vi "Test Singleton API.vi"() -> ()   [LabVIEW 2024]
doc: "Singleton API Tester."
uses:
  Singleton.lvlib
  <vilib>/Utility/error.llb/DialogType.ctl
  <vilib>/JKI/JKI Simple Localization/API/JKI Simple LocalizationJKI_Simple_Localization.lvlib
  <vilib>/JKI/JKI Simple Localization/Private/RegisterVIJKI_Simple_Localization.vi
panel:
  in  "NEW EVENT TO HL":bool
  in  "New Event":bool
  in  "Juan":bool caption="Jhon"
  out "last error":errorcluster
  in  "Show Diagram on Init":bool
  in  "wait for reply":bool=TRUE
  in  "Show Block Diagram":bool
  in  "X":dbl=1.0
  out "Reply Payload":dbl
  in  "Stop Module":bool
  in  "Start Module":bool
  out "Do Something Count":i32
  in  "Test Do Something Else and Wait for Reply":bool
  in  "Hide Module Panel":bool
  in  "Show Module Panel":bool
  in  "Test Do Something Else":bool
  in  "Test Do Something":bool
  out "Status":string
  out "Module Running?":bool
  # "This VI tests the API for the Module."
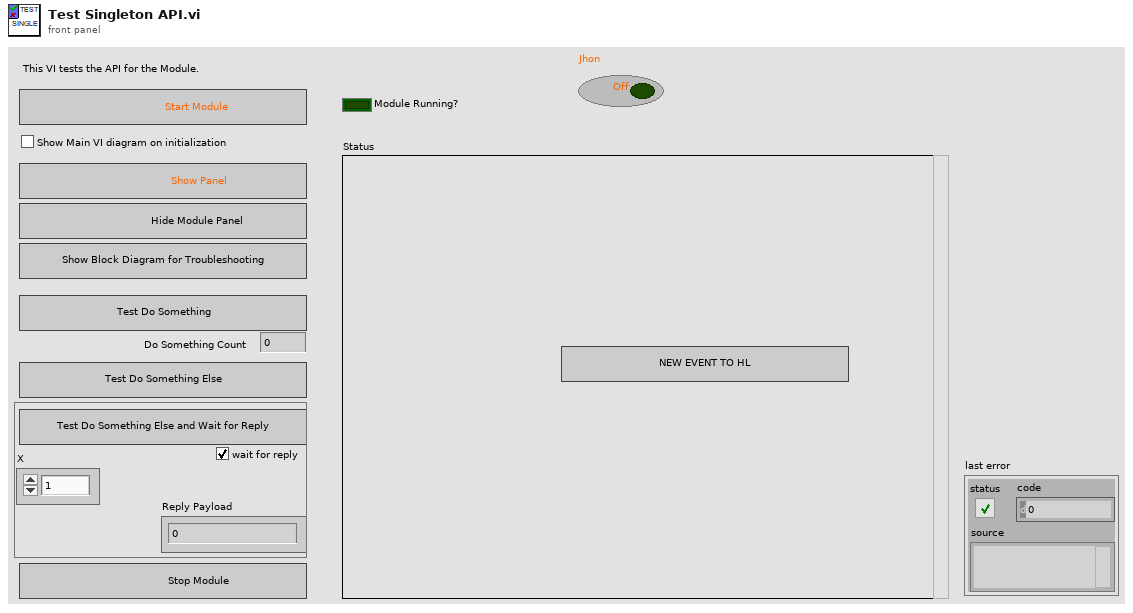
[diagram p1: front panel]
types:
  T1 = typedef "Singleton.lvlib/Broadcast Events--cluster.ctl" = cluster{"Module Did Init":refnum<user-event>, "Status Updated":refnum<user-event>, "Error Reported":refnum<user-event>, "Did Something":refnum<user-event>, "Module Did Stop":refnum<user-event>, "Update Module Execution Status":refnum<user-event>}
  T2 = typedef "DialogType.ctl" = u16
  T3 = typedef "Singleton.lvlib/Do Something Else and Wait (Reply Payload)--cluster.ctl" = cluster{"Value":dbl, "error":errorcluster}
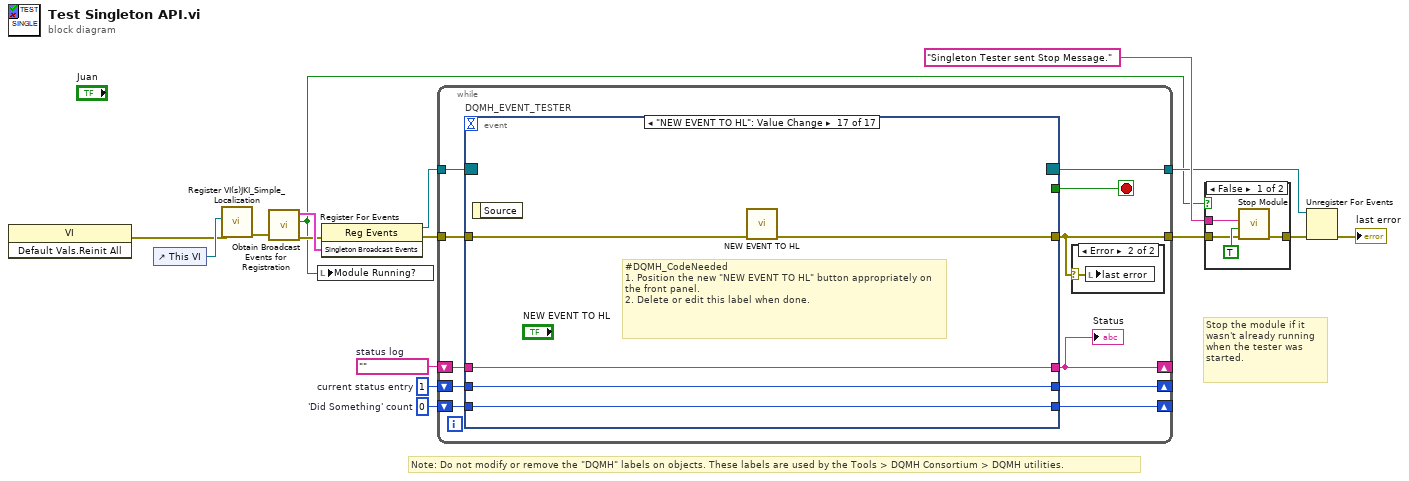
[diagram p0: block diagram]
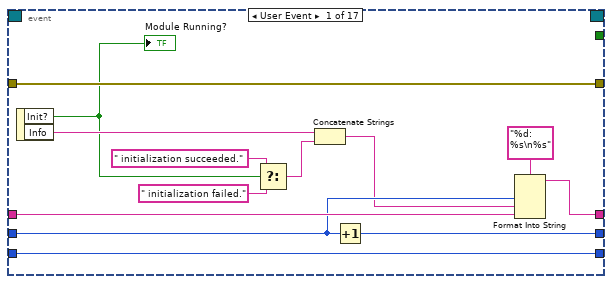
[diagram p4: hidden frame]
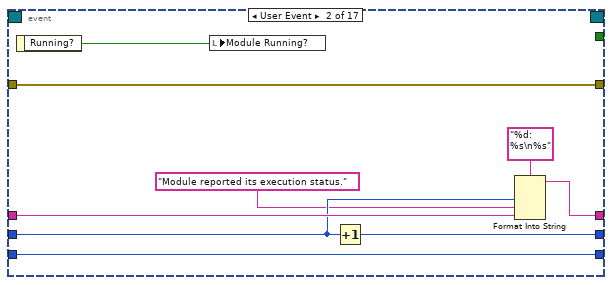
[diagram p5: hidden frame]
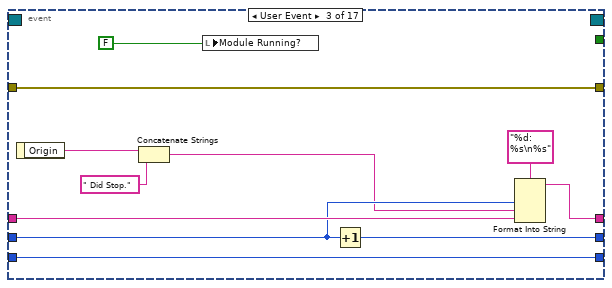
[diagram p6: hidden frame]
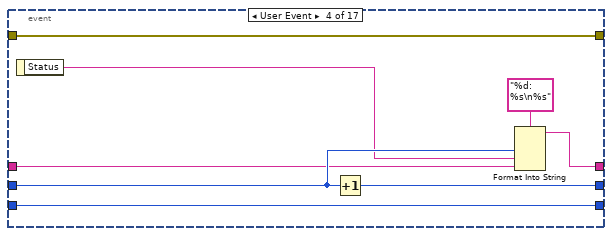
[diagram p7: hidden frame]
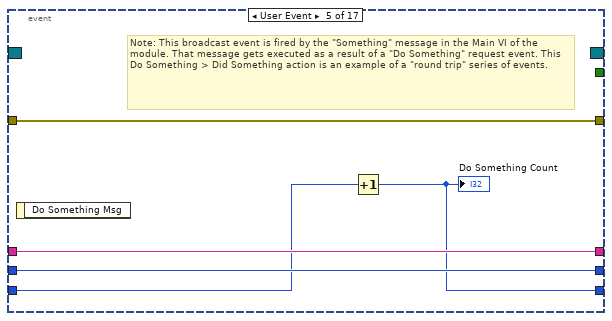
[diagram p8: hidden frame]
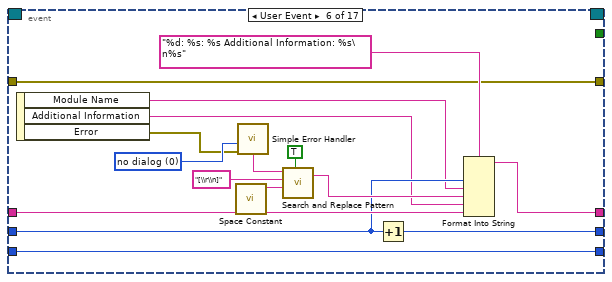
[diagram p9: hidden frame]
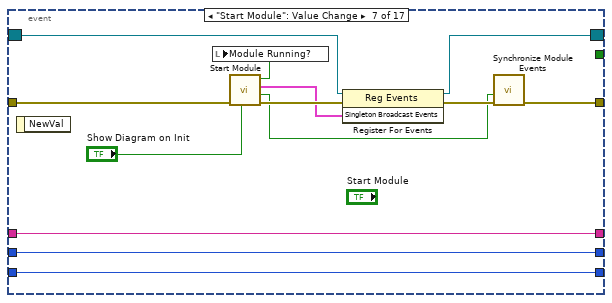
[diagram p10: hidden frame]
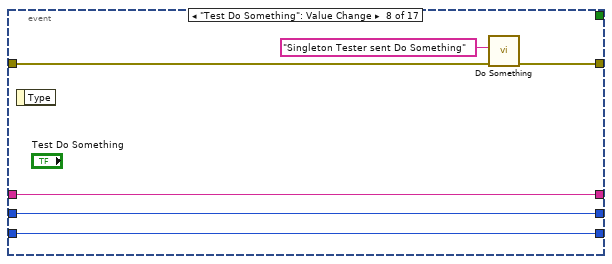
[diagram p11: hidden frame]
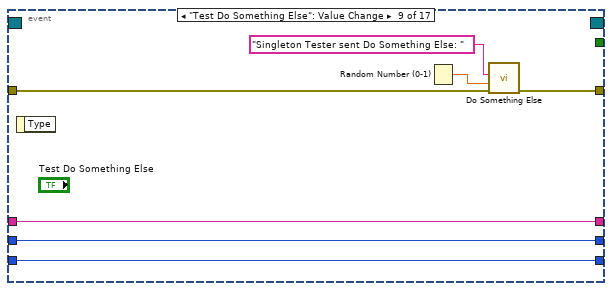
[diagram p12: hidden frame]
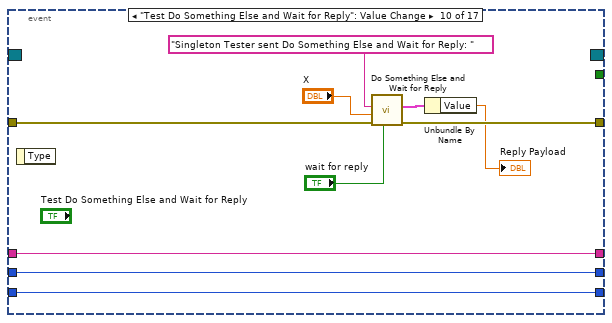
[diagram p13: hidden frame]
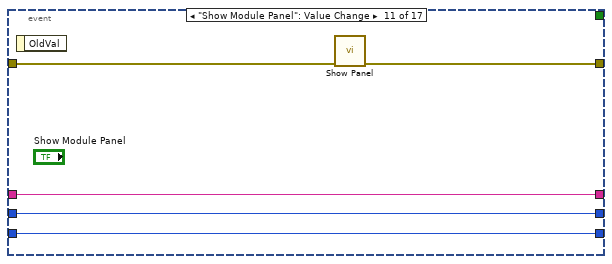
[diagram p14: hidden frame]
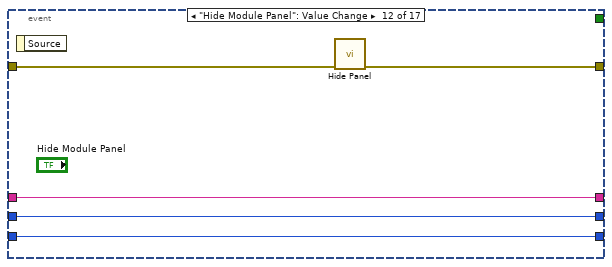
[diagram p15: hidden frame]
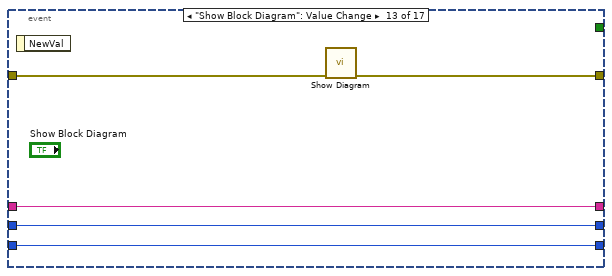
[diagram p16: hidden frame]
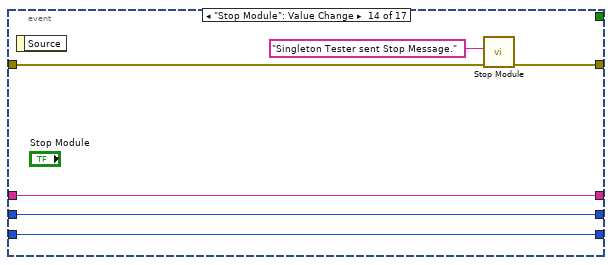
[diagram p17: hidden frame]
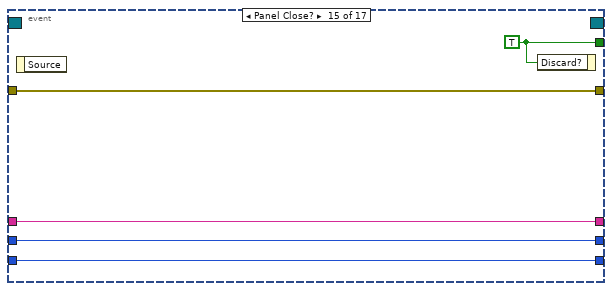
[diagram p18: hidden frame]
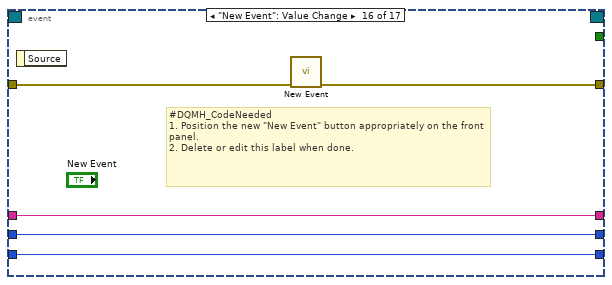
[diagram p19: hidden frame]
diagram:
  w12 = 0  # 'Did Something' count
  w13 = 1  # current status entry
  w14 = ""  # status log
  # "Stop the module if it wasn't already running when the tester was started."
  # "Note: Do not modify or remove the \"DQMH\" labels on objects. These labels are used by the Tools > DQMH Consortium > DQMH utilities."
  n1 = invoke class="VI" method="Default Vals.Reinit All"() -> (error out=w2:errorcluster)  [unwired: 3 in, 2 out]
  n2 = control-ref of="This VI"() -> (w3:refnum<vi>)
  n3 = call-poly <vilib>:"Register VI(s)JKI_Simple_Localization.vi"("error in"=w2, "VI Ref"=w3) -> ("error out"=w1:errorcluster)  [unwired: 8 in, 1 out]
  n4 = call "Obtain Broadcast Events for Registration.vi"("error in"=w1) -> ("error out"=w7:errorcluster, "Already running?"=w6:bool, "Singleton Broadcast Events"=w10:T1)  [unwired: 8 in]
  n5 = local write "Module Running?"(w6) -> ()
  n6 = register-events(error in=w7, w10) -> (reference out=w9:refnum<event-registration>, error out=w11:errorcluster)  [unwired: 1 in]
  n7 = while {
    tunnel: w9 -> [w27]
    tunnel: [w17] -> w5
    shift-right: [w23] -> _
    shift-left: w14 -> [w25]
    shift-right: [w24] -> _
    shift-left: w13 -> [w26]
    shift-right: [w21] -> _
    shift-left: w12 -> [w22]
    tunnel: w11 -> [w20]
    tunnel: [w19] -> w8
    stop <- w18 stop-if-true
    n8 = event "DQMH_EVENT_TESTER" shown="[16] \"NEW EVENT TO HL\": Value Change" {
      selector: w27 -> [_ _ _ _ _ _ w96 _ _ _ _ _ _ _ _ _ _]
      dyn-events: [_ _ _ _ _ _ w95 _ _ _ _ _ _ _ _ _ _] -> w19
      timeout: _ -> [_ _ _ _ _ _ _ _ _ _ _ _ _ _ _ _ _]
      tunnel: [_ _ _ _ _ _ _ _ _ _ _ _ _ _ w152 _ _] -> w18
      tunnel: [w41 w43 w51 w62 w70 w78 w94 w109 w116 w126 w131 w136 w137 w144 w148 w153 w158] -> w17
      tunnel: w26 -> [w38 w48 w59 w66 w73 w81 w100 w106 w112 w123 w129 w134 w139 w146 w150 w155 w160]
      tunnel: w25 -> [w39 w49 w60 w65 w74 w82 w101 w107 w113 w124 w130 w135 w140 w147 w151 w156 w161]
      tunnel: [w36 w46 w57 w67 w74 w80 w101 w107 w113 w124 w130 w135 w140 w147 w151 w156 w161] -> w23
      tunnel: [w37 w47 w58 w69 w73 w79 w100 w106 w112 w123 w129 w134 w139 w146 w150 w155 w160] -> w24
      tunnel: w22 -> [w33 w44 w53 w63 w72 w90 w99 w105 w111 w122 w128 w133 w138 w145 w149 w154 w159]
      tunnel: [w33 w44 w53 w63 w71 w90 w99 w105 w111 w122 w128 w133 w138 w145 w149 w154 w159] -> w21
      tunnel: w20 -> [w41 w43 w51 w62 w70 w78 w93 w104 w110 w119 w127 w132 w141 w142 w148 w157 w162]
      event User Event {
        n9 = event-data() -> ("Init?"=w32:bool, "Info"=w35:string)  [unwired: 1 in]
        "Module Running?" <- w32
        n10 = Select(t=" initialization succeeded.", s=w32, f=" initialization failed.") -> (s? t:f=w29:string)
        n11 = Concatenate Strings(w35, w29) -> (w34:string)
        n12 = Increment(x=w38) -> (x+1=w37:i32)
        n13 = Format Into String(format string="%d: %s\n%s", w38, w34, w39) -> (resulting string=w36:string)  [unwired: 2 in, 1 out]
      }
      event User Event {
        n14 = event-data() -> ("Running?"=w42:bool)  [unwired: 1 in]
        n15 = local write "Module Running?"(w42) -> ()
        n16 = Increment(x=w48) -> (x+1=w47:i32)
        n17 = Format Into String(format string="%d: %s\n%s", w48, "Module reported its execution status.", w49) -> (resulting string=w46:string)  [unwired: 2 in, 1 out]
      }
      event User Event {
        n18 = event-data() -> ("Origin"=w56:string)  [unwired: 1 in]
        n19 = Concatenate Strings(w56, " Did Stop.") -> (w55:string)
        n20 = local write "Module Running?"(FALSE ("Module Did Init?")) -> ()
        n21 = Increment(x=w59) -> (x+1=w58:i32)
        n22 = Format Into String(format string="%d: %s\n%s", w59, w55, w60) -> (resulting string=w57:string)  [unwired: 2 in, 1 out]
      }
      event User Event {
        n23 = event-data() -> ("Status"=w64:string)  [unwired: 1 in]
        n24 = Increment(x=w66) -> (x+1=w69:i32)
        n25 = Format Into String(format string="%d: %s\n%s", w66, w64, w65) -> (resulting string=w67:string)  [unwired: 2 in, 1 out]
      }
      event User Event {
        # "Note: This broadcast event is fired by the \"Something\" message in the Main VI of the module. That message gets executed as a result of a \"Do Something\" request event. This Do Something > Did Something action is an example of a \"round trip\" series of events."
        n26 = event-data() -> ()  [unwired: 1 in, 1 out]
        n27 = Increment(x=w72) -> (x+1=w71:i32)
        "Do Something Count" <- w71
      }
      event User Event {
        w83 = T2 0 items=["no dialog", "OK message", "continue or stop message", "OK message + warnings", "continue/stop + warnings"] ("type of dialog (OK msg:1)")
        n28 = event-data() -> ("Module Name"=w77:string, "Additional Information"=w76:string, "Error"=w75:errorcluster)  [unwired: 1 in]
        n29 = call <vilib>:"Space Constant.vi"() -> ("String"=w87:string)
        n30 = call <vilib>:"Simple Error Handler.vi"("type of dialog (OK msg:1)"=w83, "error in (no error)"=w75) -> ("message"=w84:string)  [unwired: 3 in, 4 out]
        n31 = call <vilib>:"Search and Replace Pattern.vi"("string"=w84, "regular expression (\"\")"="[\\r\\n]" ("regular expression (\"\")"), "replace string (\"\")"=w87, "replace all? (F)"=TRUE ("replace all CR/LF with spaces")) -> ("result string"=w85:string)  [unwired: 1 in, 1 out]
        n32 = Increment(x=w81) -> (x+1=w79:i32)
        n33 = Format Into String(format string="%d: %s: %s Additional Information: %s\n%s", w81, w77, w85, w76, w82) -> (resulting string=w80:string)  [unwired: 2 in, 1 out]
      }
      event "Start Module": Value Change {
        n34 = event-data() -> ()  [unwired: 1 in, 1 out]
        n35 = call "Start Module.vi"("Show Main VI Diagram on Init (F)"="Show Diagram on Init", "error in"=w93) -> ("error out"=w102:errorcluster, "Wait for Event Sync?"=w98:bool, "Singleton Broadcast Events"=w97:T1, "Module Was Already Running?"=w92:bool)  [unwired: 5 in, 1 out]
        n36 = local write "Module Running?"(w92) -> ()
        n37 = register-events(reference=w96, error in=w102, w97) -> (reference out=w95:refnum<event-registration>, error out=w103:errorcluster)
        n38 = call "Synchronize Module Events.vi"("error in"=w103, "Wait for Event Sync?"=w98) -> ("error out"=w94:errorcluster)  [unwired: 9 in]
      }
      event "Test Do Something": Value Change {
        n39 = event-data() -> ()  [unwired: 1 in, 1 out]
        n40 = call "Do Something.vi"("error in"=w104, "Do Something Message"="Singleton Tester sent Do Something") -> ("error out"=w109:errorcluster)  [unwired: 9 in]
      }
      event "Test Do Something Else": Value Change {
        n41 = event-data() -> ()  [unwired: 1 in, 1 out]
        n42 = Random Number (0-1)() -> (number: 0 to 1=w114:dbl)
        n43 = call "Do Something Else.vi"("error in"=w110, "X"=w114, "Do Something Else Message"="Singleton Tester sent Do Something Else: " ("Do Something Message")) -> ("error out"=w116:errorcluster)  [unwired: 8 in]
      }
      event "Test Do Something Else and Wait for Reply": Value Change {
        n44 = event-data() -> ()  [unwired: 1 in, 1 out]
        n45 = call "Do Something Else and Wait for Reply.vi"("wait for reply (T)"="wait for reply", "error in"=w119, "X"="X", "Do Something Else Message"="Singleton Tester sent Do Something Else and Wait for Reply: " ("Do Something Message")) -> ("error out"=w126:errorcluster, "Reply Payload"=w121:T3)  [unwired: 5 in, 1 out]
        n46 = Unbundle By Name(w121) -> ("Value"=→"Reply Payload":dbl)
      }
      event "Show Module Panel": Value Change {
        n47 = event-data() -> ()  [unwired: 1 in, 1 out]
        n48 = call "Show Panel.vi"("error in"=w127) -> ("error out"=w131:errorcluster)  [unwired: 10 in]
      }
      event "Hide Module Panel": Value Change {
        n49 = event-data() -> ()  [unwired: 1 in, 1 out]
        n50 = call "Hide Panel.vi"("error in"=w132) -> ("error out"=w136:errorcluster)  [unwired: 10 in]
      }
      event "Show Block Diagram": Value Change {
        n51 = event-data() -> ()  [unwired: 1 in, 1 out]
        n52 = call "Show Diagram.vi"("error in"=w141) -> ("error out"=w137:errorcluster)  [unwired: 10 in]
      }
      event "Stop Module": Value Change {
        n53 = event-data() -> ()  [unwired: 1 in, 1 out]
        n54 = call "Stop Module.vi"("error in"=w142, "Origin"="Singleton Tester sent Stop Message.") -> ("error out"=w144:errorcluster)  [unwired: 9 in]
      }
      event Panel Close? {
        w152 = TRUE ("Discard?")
        n55 = event-data() -> ()  [unwired: 1 in, 1 out]
        n56 = event-data("Discard?"=w152) -> ()  [unwired: 1 in, 1 out]
      }
      event "New Event": Value Change {
        # "#DQMH_CodeNeeded\n1. Position the new \"New Event\" button appropriately on the front panel.\n2. Delete or edit this label when done."
        n57 = event-data() -> ()  [unwired: 1 in, 1 out]
        n58 = call "New Event.vi"("error in"=w157) -> ("error out"=w153:errorcluster)  [unwired: 10 in]
      }
      event "NEW EVENT TO HL": Value Change {
        # "#DQMH_CodeNeeded\n1. Position the new \"NEW EVENT TO HL\" button appropriately on the front panel.\n2. Delete or edit this label when done."
        n59 = event-data() -> ()  [unwired: 1 in, 1 out]
        n60 = call "NEW EVENT TO HL.vi"("error in"=w162) -> ("error out"=w158:errorcluster)  [unwired: 10 in]
      }
    }
    "Status" <- w23
    n61 = case shown="Error" w17 {
      selector: w17 -> [_ w28]
      frame No Error {
      }
      frame Error {
        n62 = local write "last error"(w28) -> ()
      }
    }
  }
  n63 = case shown="False" w6 {
    tunnel: [w166 w167] -> w16
    tunnel: "Singleton Tester sent Stop Message." ("Origin") -> [w165 _]
    tunnel: w5 -> [w163 w167]
    frame False {
      n64 = call "Stop Module.vi"("error in"=w163, "Wait for Module to Stop? (F)"=TRUE ("Wait for Module to stop?"), "Origin"=w165) -> ("error out"=w166:errorcluster)  [unwired: 8 in]
    }
    frame True {
    }
  }
  n65 = Unregister For Events(event registration refnum=w8, error in=w16) -> (error out=→"last error":errorcluster)
